vi "SMD_soln_subvi.vi"(6 "k":dbl=2.0 format="%#_13g", 8 "b":dbl=2.0 format="%#_13g", 9 "m":dbl=2.0 format="%#_13g", 10 "Time Step":dbl=2.0 format="%#_13g", 11 "xk":dbl=2.0 format="%#_13g") -> (2 "yk":dbl, 3 "Accel":dbl)   [LabVIEW 2019]
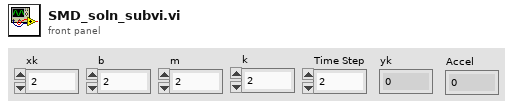
[diagram p1: front panel]
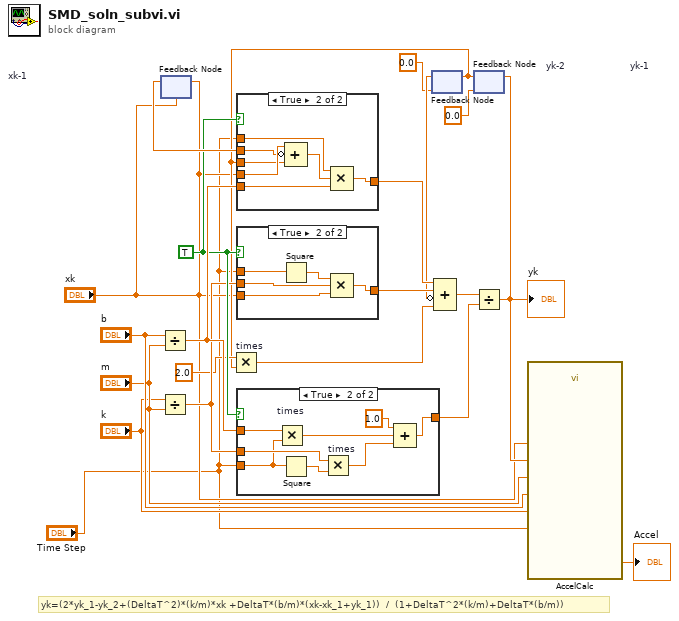
[diagram p0: block diagram]
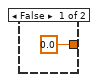
[diagram p2: hidden frame]
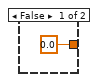
[diagram p3: hidden frame]
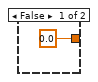
[diagram p4: hidden frame]
diagram:
  w19 = TRUE
  # "yk=(2*yk_1-yk_2+(DeltaT^2)*(k/m)*xk +DeltaT*(b/m)*(xk-xk_1+yk_1))  /  (1+DeltaT^2*(k/m)+DeltaT*(b/m))"
  n1 = Divide(x="b", y="m") -> (x/y=w21:dbl)
  n2 = Divide(x="k", y="m") -> (x/y=w18:dbl)
  n3 = feedback #1 "xk-1"("xk") -> (w20:dbl)
  n4 = feedback-in #1("xk") -> ()
  n5 = case shown="True" w19 {
    tunnel: "Time Step" -> [_ w27]
    tunnel: w18 -> [_ w25]
    tunnel: "xk" -> [_ w24]
    tunnel: [0.0 w23] -> w15
    frame False {
    }
    frame True {
      n6 = Square(x=w27) -> (x^2=w26:dbl)
      n7 = Compound Arithmetic op=MULTIPLY(w26, w25, w24) -> (w23:dbl)
    }
  }
  n8 = case shown="True" w19 {
    tunnel: "Time Step" -> [_ w29]
    tunnel: w21 -> [_ w34]
    tunnel: w18 -> [_ w32]
    tunnel: [0.0 w31] -> w17
    frame False {
    }
    frame True {
      n9 = Multiply "times"(x=w34, y=w29) -> (x*y=w35:dbl)
      n10 = Square(x=w29) -> (x^2=w30:dbl)
      n11 = Multiply "times"(x=w32, y=w30) -> (x*y=w33:dbl)
      n12 = Compound Arithmetic op=ADD(1.0 ("x"), w35, w33) -> (w31:dbl)
    }
  }
  n13 = feedback #2 "yk-2"(0.0) -> (w14:dbl)
  n14 = feedback #3 "yk-1"(0.0) -> (w12:dbl)
  n15 = Multiply "times"(x=2.0, y=w12) -> (x*y=w11:dbl)
  n16 = case shown="True" w19 {
    tunnel: "Time Step" -> [_ w39]
    tunnel: w21 -> [_ w40]
    tunnel: "xk" -> [_ w44]
    tunnel: w20 -> [_ w43]
    tunnel: w12 -> [_ w42]
    tunnel: [0.0 w38] -> w16
    frame False {
    }
    frame True {
      n17 = Compound Arithmetic op=ADD(w44, invert w43, w42) -> (w41:dbl)
      n18 = Compound Arithmetic op=MULTIPLY(w39, w41, w40) -> (w38:dbl)
    }
  }
  n19 = feedback-in #2(w12) -> ()
  n20 = Compound Arithmetic op=ADD(w16, w15, invert w14, w11) -> (w10:dbl)
  n21 = Divide(x=w10, y=w17) -> (x/y=w9:dbl)
  "yk" <- w9
  n22 = feedback-in #3(w9) -> ()
  n23 = call "AccelCalc.vi"("DeltaT"="Time Step", "yk"=w9, "k"="k", "m"="m", "b"="b", "xk"="xk") -> ("Accel 2"=→"Accel":dbl)  [unwired: 4 in, 1 out]
